vi "catalog.create_dataset.path.vi"() -> (2 "path":string)   [LabVIEW 2020, in "Nominal Client.lvclass"]
uses:
  Nominal Client.lvclass
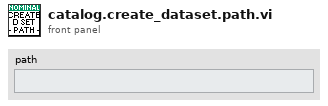
[diagram p1: front panel]
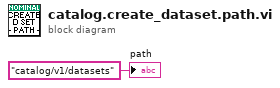
[diagram p0: block diagram]
diagram:
  "path" <- "catalog/v1/datasets" ("path")
